vi "2022_day05.vi"() -> ()   [LabVIEW 2021]
panel:
  out "Task 2":string
  out "Task 1":string
  in  "Switch":bool caption="Ex. Data  vs.  User Data"
  out "Procedure":cluster{"move":i32, "from":i32, "to":i32}[](array[cluster])
  out "Crane Stock":string[][](table)
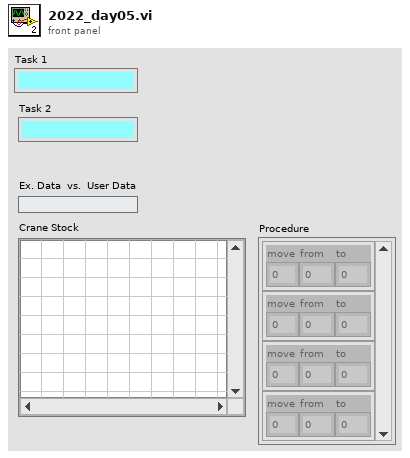
[diagram p1: front panel]
types:
  T1 = cluster{"Crane Stock":string, "Procedure":string}
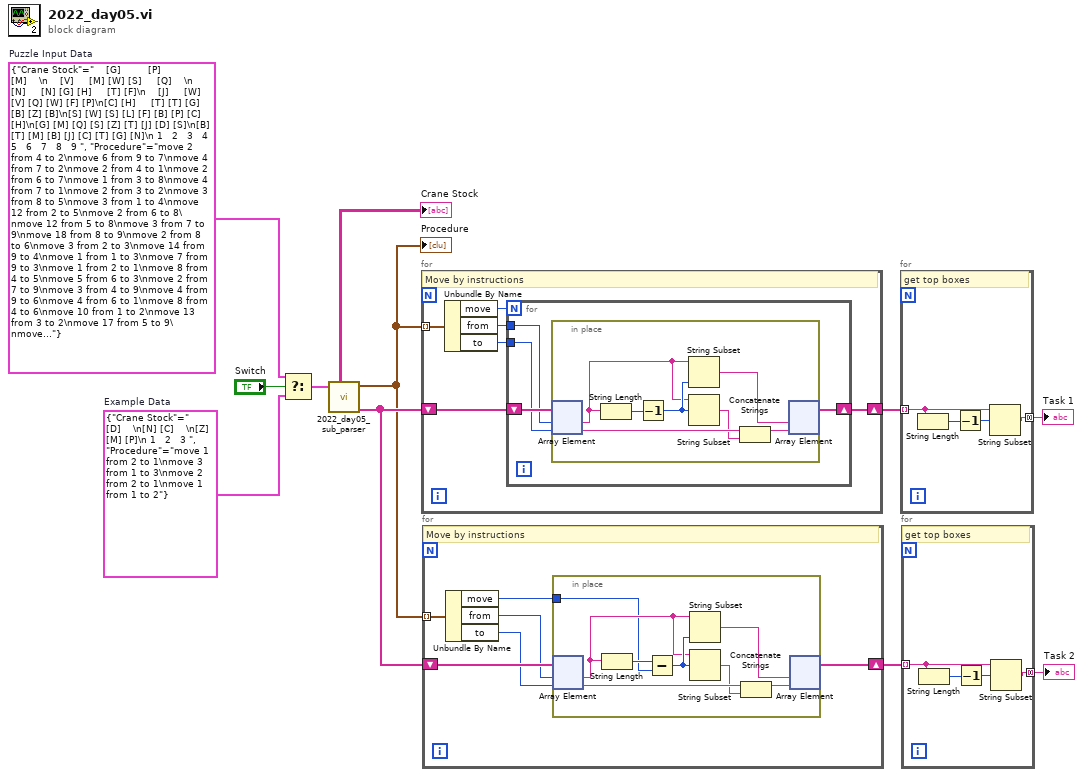
[diagram p0: block diagram]
diagram:
  w10 = T1 {"Crane Stock"="    [G]         [P]         [M]    \n    [V]     [M] [W] [S]     [Q]    \n    [N]     [N] [G] [H]     [T] [F]\n    [J]     [W] [V] [Q] [W] [F] [P]\n[C] [H]     [T] [T] [G] [B] [Z] [B]\n[S] [W] [S] [L] [F] [B] [P] [C] [H]\n[G] [M] [Q] [S] [Z] [T] [J] [D] [S]\n[B] [T] [M] [B] [J] [C] [T] [G] [N]\n 1   2   3   4   5   6   7   8   9 ", "Procedure"="move 2 from 4 to 2\nmove 6 from 9 to 7\nmove 4 from 7 to 2\nmove 2 from 4 to 1\nmove 2 from 6 to 7\nmove 1 from 3 to 8\nmove 4 from 7 to 1\nmove 2 from 3 to 2\nmove 3 from 8 to 5\nmove 3 from 1 to 4\nmove 12 from 2 to 5\nmove 2 from 6 to 8\nmove 12 from 5 to 8\nmove 3 from 7 to 9\nmove 18 from 8 to 9\nmove 2 from 8 to 6\nmove 3 from 2 to 3\nmove 14 from 9 to 4\nmove 1 from 1 to 3\nmove 7 from 9 to 3\nmove 1 from 2 to 1\nmove 8 from 4 to 5\nmove 5 from 6 to 3\nmove 2 from 7 to 9\nmove 3 from 4 to 9\nmove 4 from 9 to 6\nmove 4 from 6 to 1\nmove 8 from 4 to 6\nmove 10 from 1 to 2\nmove 13 from 3 to 2\nmove 17 from 5 to 9\nmove 2 from 5 to 1\nmove 9 from 9 to 7\nmove 1 from 3 to 6\nmove 2 from 1 to 8\nmove 11 from 2 to 4\nmove 5 from 6 to 8\nmove 1 from 6 to 3\nmove 1 from 1 to 4\nmove 3 from 8 to 6\nmove 3 from 2 to 8\nmove 9 from 7 to 9\nmove 4 from 4 to 7\nmove 1 from 9 to 5\nmove 15 from 9 to 7\nmove 7 from 8 to 3\nmove 1 from 5 to 6\nmove 2 from 6 to 9\nmove 8 from 2 to 6\nmove 3 from 4 to 3\nmove 1 from 2 to 5\nmove 4 from 9 to 3\nmove 1 from 3 to 4\nmove 13 from 6 to 2\nmove 1 from 5 to 1\nmove 4 from 4 to 9\nmove 6 from 3 to 2\nmove 11 from 2 to 7\nmove 6 from 3 to 4\nmove 3 from 3 to 2\nmove 1 from 3 to 4\nmove 1 from 1 to 3\nmove 3 from 9 to 2\nmove 1 from 3 to 1\nmove 4 from 7 to 1\nmove 1 from 9 to 5\nmove 5 from 1 to 4\nmove 11 from 2 to 4\nmove 1 from 5 to 3\nmove 1 from 2 to 3\nmove 12 from 4 to 2\nmove 2 from 7 to 2\nmove 7 from 4 to 3\nmove 5 from 4 to 1\nmove 7 from 7 to 6\nmove 4 from 1 to 8\nmove 1 from 8 to 5\nmove 8 from 3 to 2\nmove 4 from 7 to 4\nmove 13 from 7 to 1\nmove 2 from 8 to 6\nmove 5 from 4 to 9\nmove 1 from 3 to 6\nmove 1 from 5 to 8\nmove 1 from 2 to 9\nmove 4 from 2 to 6\nmove 2 from 8 to 6\nmove 10 from 1 to 3\nmove 4 from 9 to 4\nmove 2 from 1 to 3\nmove 5 from 2 to 9\nmove 4 from 9 to 2\nmove 1 from 1 to 2\nmove 13 from 2 to 4\nmove 15 from 4 to 5\nmove 3 from 6 to 8\nmove 8 from 3 to 8\nmove 1 from 4 to 2\nmove 14 from 5 to 1\nmove 1 from 5 to 4\nmove 1 from 4 to 2\nmove 8 from 6 to 7\nmove 3 from 6 to 2\nmove 2 from 9 to 1\nmove 8 from 8 to 7\nmove 9 from 1 to 5\nmove 7 from 5 to 3\nmove 14 from 7 to 9\nmove 2 from 2 to 3\nmove 7 from 2 to 1\nmove 1 from 6 to 1\nmove 4 from 9 to 2\nmove 8 from 3 to 6\nmove 2 from 4 to 3\nmove 4 from 3 to 5\nmove 5 from 5 to 7\nmove 2 from 6 to 9\nmove 6 from 6 to 2\nmove 4 from 2 to 3\nmove 1 from 6 to 2\nmove 2 from 7 to 8\nmove 13 from 9 to 5\nmove 2 from 7 to 1\nmove 14 from 1 to 5\nmove 15 from 5 to 7\nmove 3 from 8 to 7\nmove 5 from 3 to 5\nmove 6 from 5 to 7\nmove 4 from 1 to 7\nmove 1 from 2 to 5\nmove 3 from 2 to 8\nmove 11 from 5 to 2\nmove 10 from 7 to 1\nmove 1 from 3 to 4\nmove 10 from 2 to 9\nmove 1 from 5 to 8\nmove 6 from 7 to 3\nmove 1 from 4 to 6\nmove 2 from 3 to 8\nmove 1 from 2 to 1\nmove 4 from 3 to 9\nmove 3 from 1 to 6\nmove 2 from 7 to 1\nmove 1 from 5 to 6\nmove 1 from 3 to 8\nmove 4 from 1 to 4\nmove 5 from 2 to 9\nmove 3 from 1 to 4\nmove 18 from 9 to 7\nmove 4 from 8 to 4\nmove 3 from 1 to 2\nmove 1 from 9 to 7\nmove 1 from 4 to 7\nmove 1 from 6 to 2\nmove 1 from 2 to 5\nmove 25 from 7 to 3\nmove 7 from 4 to 2\nmove 8 from 7 to 9\nmove 4 from 8 to 6\nmove 1 from 8 to 5\nmove 4 from 6 to 5\nmove 2 from 9 to 5\nmove 3 from 5 to 8\nmove 4 from 6 to 4\nmove 12 from 3 to 5\nmove 11 from 3 to 2\nmove 13 from 5 to 8\nmove 4 from 9 to 6\nmove 7 from 4 to 9\nmove 2 from 6 to 2\nmove 12 from 2 to 7\nmove 1 from 6 to 3\nmove 1 from 5 to 6\nmove 2 from 5 to 3\nmove 15 from 8 to 6\nmove 4 from 6 to 7\nmove 1 from 5 to 1\nmove 10 from 2 to 8\nmove 8 from 8 to 3\nmove 8 from 6 to 8\nmove 2 from 7 to 6\nmove 9 from 9 to 7\nmove 8 from 8 to 9\nmove 1 from 1 to 3\nmove 1 from 2 to 7\nmove 7 from 3 to 1\nmove 3 from 8 to 5\nmove 3 from 1 to 6\nmove 7 from 9 to 2\nmove 2 from 3 to 7\nmove 5 from 7 to 9\nmove 17 from 7 to 5\nmove 2 from 7 to 6\nmove 10 from 6 to 3\nmove 1 from 1 to 3\nmove 6 from 9 to 3\nmove 1 from 2 to 9\nmove 2 from 7 to 9\nmove 2 from 9 to 7\nmove 1 from 5 to 8\nmove 1 from 8 to 5\nmove 6 from 2 to 5\nmove 1 from 6 to 1\nmove 5 from 3 to 5\nmove 1 from 6 to 8\nmove 1 from 7 to 9\nmove 2 from 9 to 3\nmove 15 from 5 to 2\nmove 2 from 1 to 8\nmove 2 from 3 to 7\nmove 2 from 8 to 3\nmove 3 from 5 to 9\nmove 1 from 8 to 6\nmove 1 from 9 to 6\nmove 3 from 7 to 6\nmove 17 from 3 to 4\nmove 1 from 1 to 2\nmove 6 from 2 to 9\nmove 16 from 4 to 1\nmove 4 from 6 to 8\nmove 9 from 5 to 6\nmove 8 from 6 to 2\nmove 2 from 9 to 5\nmove 2 from 3 to 5\nmove 1 from 6 to 2\nmove 1 from 4 to 8\nmove 14 from 1 to 3\nmove 8 from 5 to 3\nmove 20 from 3 to 1\nmove 1 from 8 to 2\nmove 1 from 9 to 6\nmove 1 from 6 to 7\nmove 1 from 7 to 3\nmove 22 from 1 to 2\nmove 3 from 3 to 6\nmove 27 from 2 to 8\nmove 2 from 2 to 8\nmove 2 from 6 to 9\nmove 2 from 9 to 4\nmove 2 from 4 to 8\nmove 1 from 1 to 3\nmove 14 from 8 to 5\nmove 1 from 3 to 9\nmove 3 from 9 to 2\nmove 5 from 2 to 8\nmove 10 from 2 to 9\nmove 1 from 6 to 7\nmove 1 from 7 to 5\nmove 7 from 5 to 2\nmove 2 from 9 to 2\nmove 1 from 6 to 2\nmove 2 from 9 to 5\nmove 3 from 5 to 6\nmove 6 from 5 to 3\nmove 1 from 5 to 6\nmove 4 from 3 to 9\nmove 2 from 9 to 8\nmove 3 from 9 to 5\nmove 23 from 8 to 1\nmove 2 from 6 to 1\nmove 1 from 5 to 7\nmove 2 from 3 to 5\nmove 2 from 9 to 5\nmove 4 from 9 to 7\nmove 2 from 9 to 4\nmove 1 from 5 to 4\nmove 5 from 8 to 5\nmove 2 from 6 to 2\nmove 3 from 7 to 3\nmove 1 from 3 to 4\nmove 3 from 2 to 8\nmove 4 from 1 to 6\nmove 2 from 6 to 3\nmove 4 from 1 to 2\nmove 3 from 8 to 1\nmove 13 from 2 to 5\nmove 4 from 3 to 2\nmove 14 from 5 to 7\nmove 5 from 2 to 7\nmove 18 from 7 to 9\nmove 4 from 4 to 7\nmove 2 from 5 to 4\nmove 17 from 9 to 5\nmove 1 from 9 to 1\nmove 1 from 7 to 2\nmove 5 from 7 to 2\nmove 18 from 1 to 4\nmove 1 from 7 to 3\nmove 1 from 3 to 6\nmove 2 from 1 to 3\nmove 1 from 6 to 5\nmove 2 from 6 to 8\nmove 1 from 8 to 9\nmove 1 from 8 to 3\nmove 13 from 4 to 5\nmove 1 from 1 to 6\nmove 3 from 2 to 4\nmove 1 from 6 to 1\nmove 3 from 2 to 9\nmove 3 from 3 to 1\nmove 5 from 4 to 5\nmove 30 from 5 to 3\nmove 1 from 4 to 6\nmove 1 from 9 to 8\nmove 1 from 9 to 6\nmove 21 from 3 to 7\nmove 3 from 1 to 6\nmove 1 from 1 to 4\nmove 1 from 9 to 6\nmove 1 from 8 to 2\nmove 1 from 3 to 6\nmove 1 from 9 to 3\nmove 5 from 4 to 8\nmove 1 from 2 to 4\nmove 9 from 5 to 7\nmove 2 from 5 to 9\nmove 2 from 8 to 2\nmove 2 from 6 to 3\nmove 1 from 4 to 1\nmove 4 from 3 to 8\nmove 2 from 9 to 2\nmove 4 from 2 to 6\nmove 1 from 1 to 4\nmove 2 from 6 to 9\nmove 2 from 5 to 4\nmove 1 from 3 to 1\nmove 1 from 1 to 3\nmove 2 from 9 to 1\nmove 5 from 3 to 5\nmove 1 from 1 to 8\nmove 4 from 6 to 4\nmove 5 from 5 to 6\nmove 18 from 7 to 5\nmove 1 from 3 to 4\nmove 12 from 7 to 5\nmove 15 from 5 to 6\nmove 1 from 5 to 8\nmove 1 from 3 to 7\nmove 1 from 1 to 2\nmove 1 from 2 to 4\nmove 1 from 7 to 9\nmove 2 from 8 to 2\nmove 1 from 2 to 4\nmove 4 from 4 to 2\nmove 1 from 2 to 1\nmove 1 from 9 to 8\nmove 4 from 6 to 4\nmove 3 from 2 to 6\nmove 1 from 2 to 6\nmove 8 from 4 to 3\nmove 1 from 1 to 3\nmove 6 from 6 to 1\nmove 1 from 3 to 6\nmove 5 from 1 to 7\nmove 10 from 5 to 9\nmove 3 from 9 to 8\nmove 7 from 6 to 2\nmove 1 from 7 to 8\nmove 3 from 5 to 8\nmove 3 from 6 to 2\nmove 6 from 8 to 9\nmove 1 from 5 to 3\nmove 2 from 3 to 1\nmove 2 from 4 to 8\nmove 6 from 6 to 9\nmove 1 from 1 to 4\nmove 17 from 9 to 2\nmove 1 from 4 to 1\nmove 2 from 7 to 8\nmove 1 from 9 to 8\nmove 3 from 8 to 4\nmove 3 from 1 to 4\nmove 9 from 8 to 2\nmove 1 from 8 to 4\nmove 12 from 2 to 7\nmove 4 from 7 to 4\nmove 1 from 8 to 1\nmove 10 from 4 to 2\nmove 3 from 3 to 2\nmove 1 from 9 to 7\nmove 11 from 7 to 3\nmove 1 from 3 to 1\nmove 2 from 3 to 9\nmove 1 from 3 to 7\nmove 2 from 1 to 9\nmove 1 from 6 to 5\nmove 7 from 3 to 6\nmove 1 from 7 to 3\nmove 3 from 3 to 4\nmove 1 from 5 to 7\nmove 2 from 4 to 3\nmove 2 from 4 to 8\nmove 1 from 7 to 6\nmove 2 from 6 to 8\nmove 1 from 9 to 2\nmove 1 from 9 to 5\nmove 1 from 5 to 1\nmove 1 from 8 to 6\nmove 1 from 3 to 2\nmove 4 from 6 to 1\nmove 5 from 1 to 4\nmove 11 from 2 to 4\nmove 2 from 8 to 2\nmove 1 from 8 to 9\nmove 27 from 2 to 5\nmove 4 from 6 to 3\nmove 3 from 2 to 4\nmove 2 from 5 to 9\nmove 1 from 5 to 7\nmove 2 from 9 to 5\nmove 14 from 4 to 7\nmove 2 from 4 to 7\nmove 3 from 4 to 8\nmove 4 from 3 to 1\nmove 4 from 1 to 8\nmove 2 from 3 to 9\nmove 2 from 9 to 3\nmove 7 from 8 to 9\nmove 1 from 3 to 8\nmove 2 from 3 to 2\nmove 25 from 5 to 9\nmove 1 from 5 to 8\nmove 1 from 8 to 7\nmove 26 from 9 to 1\nmove 23 from 1 to 5\nmove 7 from 9 to 7\nmove 1 from 9 to 8\nmove 1 from 9 to 2\nmove 5 from 7 to 1\nmove 20 from 5 to 6\nmove 1 from 7 to 6\nmove 2 from 5 to 3\nmove 1 from 8 to 6\nmove 21 from 6 to 8\nmove 1 from 6 to 4\nmove 1 from 1 to 7\nmove 2 from 1 to 6\nmove 1 from 1 to 3\nmove 1 from 2 to 5\nmove 1 from 2 to 6\nmove 2 from 7 to 6\nmove 6 from 7 to 9\nmove 3 from 1 to 2\nmove 17 from 8 to 1\nmove 1 from 4 to 1\nmove 2 from 6 to 9\nmove 3 from 8 to 9\nmove 2 from 3 to 7\nmove 2 from 9 to 8\nmove 4 from 7 to 3\nmove 4 from 3 to 4\nmove 2 from 5 to 8\nmove 4 from 8 to 4\nmove 3 from 6 to 8\nmove 18 from 1 to 5\nmove 1 from 3 to 4\nmove 3 from 2 to 4\nmove 5 from 9 to 1\nmove 10 from 7 to 5\nmove 5 from 1 to 3\nmove 5 from 3 to 5\nmove 5 from 4 to 3\nmove 2 from 4 to 2\nmove 5 from 8 to 3\nmove 25 from 5 to 2\nmove 3 from 3 to 6\nmove 1 from 1 to 3\nmove 3 from 6 to 7\nmove 1 from 4 to 2\nmove 1 from 5 to 8\nmove 2 from 4 to 9\nmove 1 from 8 to 1\nmove 20 from 2 to 7\nmove 10 from 7 to 1\nmove 1 from 1 to 7\nmove 4 from 7 to 8\nmove 5 from 5 to 4\nmove 4 from 8 to 6\nmove 1 from 1 to 3\nmove 5 from 7 to 4\nmove 2 from 1 to 5\nmove 4 from 9 to 1\nmove 3 from 2 to 5\nmove 5 from 5 to 1\nmove 1 from 9 to 1\nmove 11 from 1 to 3\nmove 1 from 6 to 2\nmove 7 from 3 to 5\nmove 11 from 3 to 7\nmove 1 from 2 to 6\nmove 7 from 7 to 8\nmove 1 from 9 to 1\nmove 2 from 3 to 1\nmove 1 from 5 to 3\nmove 4 from 1 to 6\nmove 4 from 6 to 3\nmove 9 from 4 to 5\nmove 2 from 8 to 2\nmove 4 from 6 to 9\nmove 3 from 2 to 4\nmove 1 from 8 to 6"}  # Puzzle Input Data
  w9 = T1 {"Crane Stock"="    [D]    \n[N] [C]    \n[Z] [M] [P]\n 1   2   3 ", "Procedure"="move 1 from 2 to 1\nmove 3 from 1 to 3\nmove 2 from 2 to 1\nmove 1 from 1 to 2"}  # Example Data
  n1 = Select(t=w10, s="Switch", f=w9) -> (s? t:f=w11:T1)
  n2 = call "2022_day05_sub_parser.vi"("Data"=w11) -> ("Crane Stock (for Algorithm)"=w2:string[], "Rearrangement Procedure"=w1:cluster{"move":i32, "from":i32, "to":i32}[], "Crane Stock (Table)"=→"Crane Stock":string[][])  [unwired: 8 in]
  "Procedure" <- w1
  n3 = for {
    tunnel: w1 -> [w14] mode=indexing
    shift-right: [w16] -> w7
    shift-left: w2 -> [w17]
    # "Move by instructions"
    n4 = Unbundle By Name(w14) -> ("move"=w15:i32, "from"=w13:i32, "to"=w12:i32)
    n5 = for {
      N: w15 -> [_]
      shift-right: [w18] -> w16
      shift-left: w17 -> [w21]
      tunnel: w13 -> [w20]
      tunnel: w12 -> [w19]
      n6 = in-place {
        n7 = in-place-array #1(w21, w20, w19) -> (w23:string, w28:string)
        n8 = String Length(string=w23) -> (length=w25:i32)
        n9 = Decrement(x=w25) -> (x-1=w24:i32)
        n10 = String Subset(string=w23, length (rest)=w24) -> (substring=w22:string)  [unwired: 1 in]
        n11 = String Subset(string=w23, offset (0)=w24) -> (substring=w26:string)  [unwired: 1 in]
        n12 = Concatenate Strings(w28, w26) -> (w27:string)
        n13 = in-place-array #1(w22, w27) -> (w18:string[])  [unwired: 2 out]
      }
    }
  }
  n14 = for {
    tunnel: w1 -> [w32] mode=indexing
    shift-right: [w33] -> w4
    shift-left: w2 -> [w34]
    # "Move by instructions"
    n15 = Unbundle By Name(w32) -> ("move"=w29:i32, "from"=w31:i32, "to"=w30:i32)
    n16 = in-place {
      in-place-border: w29 -> [w35]
      n17 = in-place-array #2(w34, w31, w30) -> (w37:string, w42:string)
      n18 = String Length(string=w37) -> (length=w39:i32)
      n19 = Subtract(x=w39, y=w35) -> (x-y=w38:i32)
      n20 = String Subset(string=w37, length (rest)=w38) -> (substring=w36:string)  [unwired: 1 in]
      n21 = String Subset(string=w37, offset (0)=w38) -> (substring=w40:string)  [unwired: 1 in]
      n22 = Concatenate Strings(w42, w40) -> (w41:string)
      n23 = in-place-array #2(w36, w41) -> (w33:string[])  [unwired: 2 out]
    }
  }
  n24 = for {
    tunnel: w7 -> [w44] mode=indexing
    tunnel: [w43] -> w6 mode=concatenating
    # "get top boxes"
    n25 = String Length(string=w44) -> (length=w45:i32)
    n26 = Decrement(x=w45) -> (x-1=w46:i32)
    n27 = String Subset(string=w44, offset (0)=w46) -> (substring=w43:string)  [unwired: 1 in]
  }
  "Task 1" <- w6
  n28 = for {
    tunnel: w4 -> [w48] mode=indexing
    tunnel: [w47] -> w5 mode=concatenating
    # "get top boxes"
    n29 = String Length(string=w48) -> (length=w49:i32)
    n30 = Decrement(x=w49) -> (x-1=w50:i32)
    n31 = String Subset(string=w48, offset (0)=w50) -> (substring=w47:string)  [unwired: 1 in]
  }
  "Task 2" <- w5
